vi "Filter Only Zombies.vi"(8 "Error In":errorcluster, 11 "All Bookmarks":T2) -> (0 "Error Out":errorcluster, 3 "Zombies":T1(array[cluster]))   [LabVIEW 2017, in "Graveyard.lvlib"]
doc: "Filters out all bookmarks that are NOT zombies"
uses:
  Graveyard.lvlib
  <vilib>/Utility/miscctls.llb/LVBookmarkInfoTypeDef.ctl
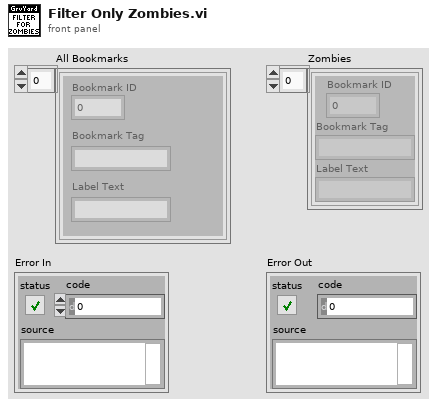
[diagram p1: front panel]
types:
  T1 = cluster{"Bookmark ID":u32, "Bookmark Tag":string, "Label Text":string}[]
  T2 = typedef "LVBookmarkInfoTypeDef.ctl" = cluster{"Bookmark ID":u32, "Bookmark Tag":string, "Label Text":string}[]
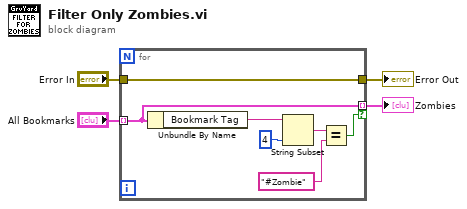
[diagram p0: block diagram]
diagram:
  n1 = for {
    tunnel: "All Bookmarks" -> [w7] mode=indexing
    tunnel: [w7] -> w3 mode=indexing if=w5
    tunnel: "Error In" -> [w6]
    tunnel: [w6] -> w1
    n2 = Unbundle By Name(w7) -> ("Bookmark Tag"=w8:string)
    n3 = String Subset(string=w8, length (rest)=4 ("length (rest)")) -> (substring=w10:string)  [unwired: 1 in]
    n4 = Equal?(x=w10, y="#Zombie") -> (x = y?=w5:bool)
  }
  "Zombies" <- w3
  "Error Out" <- w1
